vi "AutoSetXZ.vi"(8 "error in (no error)":errorcluster, 9 "SetZ":dbl, 10 "SetY":dbl, 11 "SetX":dbl) -> (0 "error out":errorcluster)   [LabVIEW 2020]
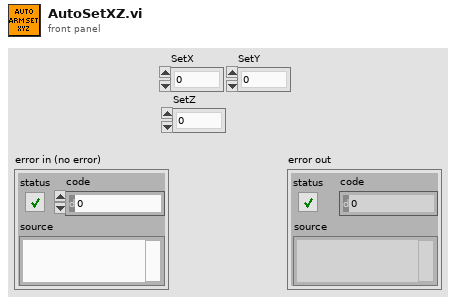
[diagram p1: front panel]
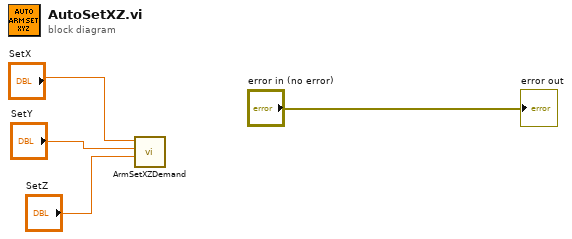
[diagram p0: block diagram]
diagram:
  n1 = call "ArmSetXZDemand.vi"("SetZ"="SetZ", 10:"SetY", "SetX"="SetX") -> ()  [unwired: 9 in]
  "error out" <- "error in (no error)"
